vi "3C Helper - Convert Given Values To PWM.vi"(11 "Setpoints to boat":T1) -> (2 "Output Array, integers":u8[](array[numeric]), 3 "output array":T3[](array[typedef]))   [LabVIEW 2011]
uses:
  2-RIO/2 Typedefs/rudder angle.ctl
  2-RIO/2 Typedefs/setpoints to boat.ctl
  2-RIO/2 Typedefs/sail setpt.ctl
panel:
  # "Control from the global variable"
  # "Indicator of Output Array"
  # "Output Array"
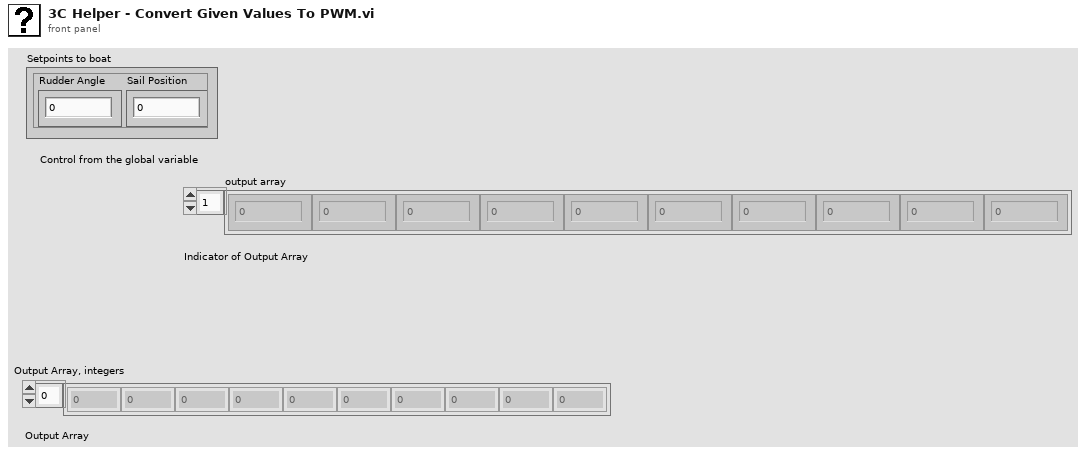
[diagram p1: front panel]
types:
  T1 = typedef "setpoints to boat.ctl" = cluster{"Sail Position":T2, "Rudder Angle":T3}
  T2 = typedef "sail setpt.ctl" = dbl
  T3 = typedef "rudder angle.ctl" = dbl
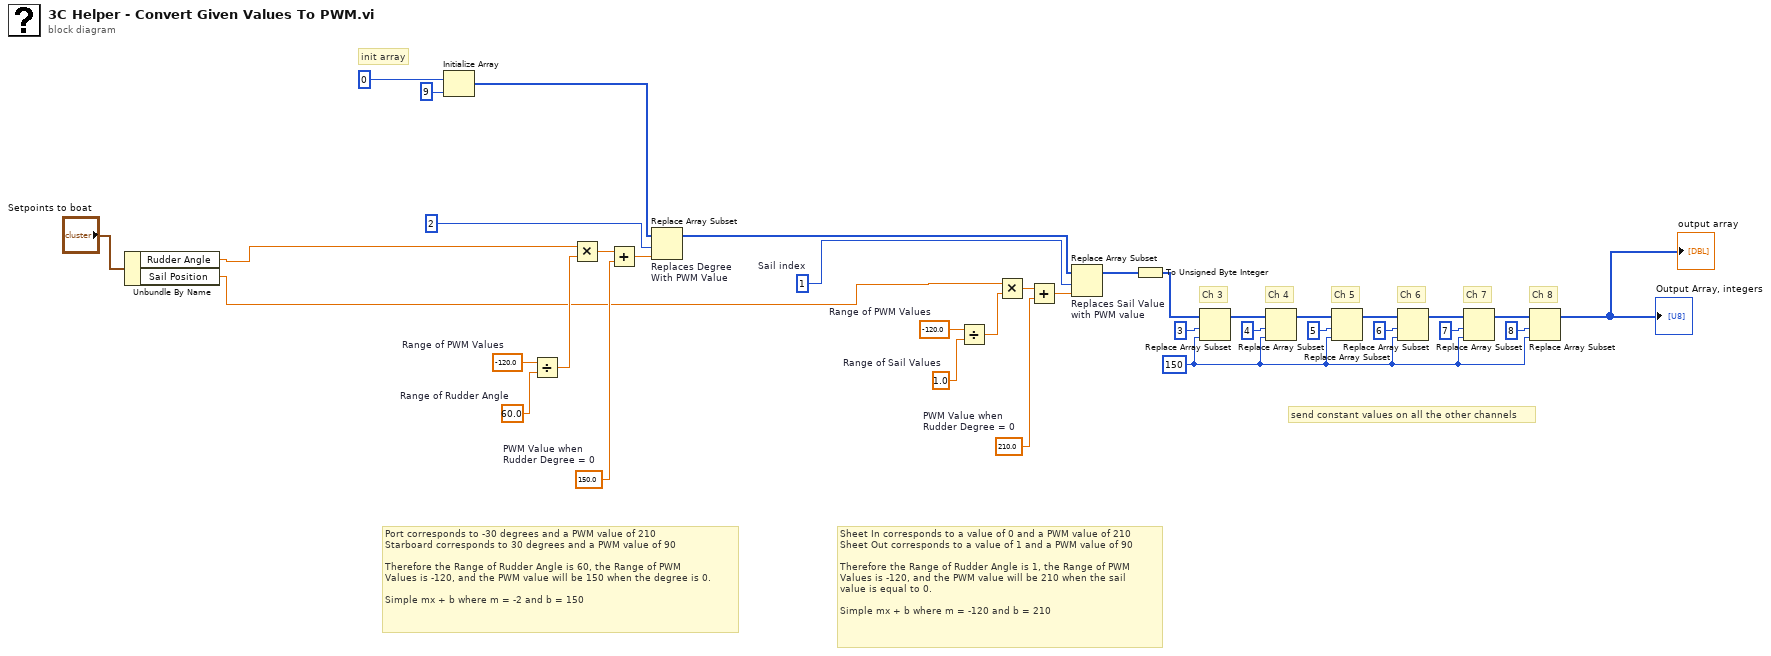
[diagram p0: block diagram]
diagram:
  w10 = u8 150
  w36 = T3 210.0  # PWM Value when Rudder Degree = 0
  w32 = 1.0  # Range of Sail Values
  w31 = -120.0  # Range of PWM Values
  w29 = T3 150.0  # PWM Value when Rudder Degree = 0
  w26 = 60.0  # Range of Rudder Angle
  w25 = -120.0  # Range of PWM Values
  w24 = 1  # Sail index
  # "init array"
  # "send constant values on all the other channels"
  # "Ch 8"
  # "Ch 7"
  # "Ch 6"
  # "Ch 5"
  # "Ch 4"
  # "Ch 3"
  # "Sheet In corresponds to a value of 0 and a PWM value of 210\nSheet Out corresponds to a value of 1 and a PWM value of 90\n\nTherefore the Range of Rudder Angle is 1, the Range of PWM\nValues is -120, and the PWM value will be 210 when the sail\nvalue is equal to 0.\n\nSimple mx + b where m = -120 and b = 210"
  # "Port corresponds to -30 degrees and a PWM value of 210\nStarboard corresponds to 30 degrees and a PWM value of 90\n\nTherefore the Range of Rudder Angle is 60, the Range of PWM\nValues is -120, and the PWM value will be 150 when the degree is 0.\n\nSimple mx + b where m = -2 and b = 150"
  n1 = Unbundle By Name("Setpoints to boat") -> ("Rudder Angle"=w2:T3, "Sail Position"=w3:T2)
  n2 = Initialize Array(u8 0 ("element"), 9 ("dimension size")) -> (w5:u8[])
  n3 = Divide(x=w25, y=w26) -> (x/y=w27:dbl)
  n4 = Multiply(x=w2, y=w27) -> (x*y=w28:T3)
  n5 = Add(x=w28, y=w29) -> (x+y=w30:T3)
  n6 = Replace Array Subset "Replaces Degree\nWith PWM Value"(array=w5, new element=w30, index=2) -> (w23:u8[])
  n7 = Divide(x=w31, y=w32) -> (x/y=w33:dbl)
  n8 = Multiply(x=w3, y=w33) -> (x*y=w34:T2)
  n9 = Add(x=w34, y=w36) -> (x+y=w35:T2)
  n10 = Replace Array Subset "Replaces Sail Value\nwith PWM value"(array=w23, new element=w35, index=w24) -> (w22:u8[])
  n11 = To Unsigned Byte Integer(number=w22) -> (unsigned 8bit integer=w9:u8[])
  n12 = Replace Array Subset(array=w9, new element=w10, index=3) -> (w19:u8[])
  n13 = Replace Array Subset(array=w19, new element=w10, index=4) -> (w17:u8[])
  n14 = Replace Array Subset(array=w17, new element=w10, index=5) -> (w15:u8[])
  n15 = Replace Array Subset(array=w15, new element=w10, index=6) -> (w13:u8[])
  n16 = Replace Array Subset(array=w13, new element=w10, index=7) -> (w11:u8[])
  n17 = Replace Array Subset(array=w11, new element=w10, index=8) -> (→"output array" →"Output Array, integers":u8[])
